vi "PH_HamamatsuCamera.PC set Right.vi"(0 "i ref in":refnum<vi>, 1 "No Info? (False)":bool, 2 "Right":u32, 3 "Maximum Right":u32, 4 "Minimum Right":u32, 5 "error in (no error)":errorcluster, 7 "Right writable? (True)":bool=TRUE) -> (14 "i ref out":refnum<vi>, 17 "Right changed?":bool, 19 "error out":errorcluster)   [LabVIEW 2014]
doc: "This VI sets the incoming value to own attributes and the GUI element."
uses:
  PH_HamamatsuCamera.lvlib
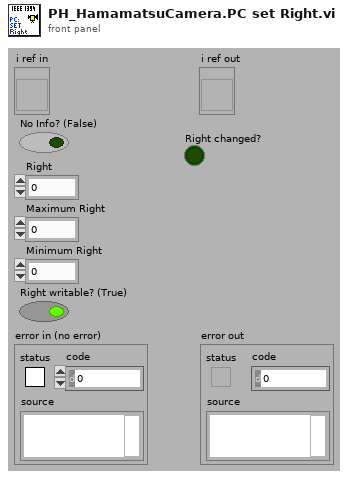
[diagram p1: front panel]
types:
  T1 = enum8{"Enabled", "Disabled", "Disabled and Grayed Out"}
  T2 = typedef "PH_HamamatsuCamera.lvlib/PH_HamamatsuCamera.i attribute.ctl" = cluster{"Gui Refs":cluster{"Frame Rate":refnum<vi>, "Get Frame Rate":refnum<vi>, "Camera State":refnum<vi>, "Start Cam":refnum<vi>, "Show Image":refnum<vi>, "Get Histogram":refnum<vi>, "Mapping":refnum<vi>, "Histogram":refnum<vi>, "Center Cross":refnum<vi>, "Center of Gravity":refnum<vi>, "Scale Factor [%]":refnum<vi>, "Save Image":refnum<vi>, "Palette":refnum<vi>, "Connect":refnum<vi>, "Camera State Bar":refnum<vi>, "Cam Error":refnum<vi>, "Camera Details":refnum<vi>, "ROI":refnum<vi>, "Set ROI to Maximum":refnum<vi>, "Trigger Parameters":refnum<vi>, "Brightness":refnum<vi>, "Shutter":refnum<vi>, "Gain":refnum<vi>, "Trigger Timeout":refnum<vi>, "Subtract Background":refnum<vi>, "Cam List":refnum<vi>, "Parameters":refnum<vi>, "Trigger Polarity":refnum<vi>, "Trigger Mode":refnum<vi>}, "Cam":cluster{"State":T3, "Restart":bool, "Source Notifier":refnum<notifier>, "Handle":i32, "Details":cluster{"Model":string, "Camera ID":string, "Firmware":string}, "Error":errorcluster, "Buffer Info":cluster{"height":u32, "width":u32, "datatype":u32}}, "Images":cluster{"CamI16":T4, "OperationI16":T4, "PSDB I16":T4}, "Window Image":cluster{"Indicate Image":bool, "Window No.":i32, "Scale Facor":dbl, "Center Cross":bool, "Subtract Backgr":bool, "CoG":bool, "Color Palette":cluster{"Red":u8, "Green":u8, "Blue":u8}[], "Image On":bool}, "Default Prdc Int":i32, "Performance":cluster{"on":bool, "Timestamp Last Frame":i32}, "Histogram":cluster{"on":bool, "Mapping":bool}, "Save Image":cluster{"Save":bool, "File refnum":refnum<file>}, "Setting Service ID":i32, "GUI Manager Path":string, "Screen":cluster{"x-resolution":i16, "y-resolution":i16}, "Image Position Path":string, "H Offset":cluster{"Value":i32, "Minimum":i32, "Maximum":i32, "Increment":i32}, "V Offset":cluster{"Value":i32, "Minimum":i32, "Maximum":i32, "Increment":i32}, "H Width":cluster{"Value":i32, "Minimum":i32, "Maximum":i32, "Increment":i32}, "V Width":cluster{"Value":i32, "Minimum":i32, "Maximum":i32, "Increment":i32}, "Trigger Parameters":cluster{"Mode":u32, "Polarity":u32, "Times":u32, "Delay":dbl}, "Trigger Timeout":u32, "Parameters":T5[], "Cam Setting Parameters":cluster{"Brightness":string, "Shutter":string, "Gain":string}}
  T3 = typedef "Device State.ctl" = i32
  T4 = typedef "IMAQ Image.ctl" = refnum<image>
  T5 = typedef "PH_HamamatsuCamera.lvlib/PH_HamamatsuCamera.Parameter Set.ctl" = cluster{"Name":string, "Value":dbl, "Range":cluster{"min":dbl, "max":dbl, "step":dbl}}
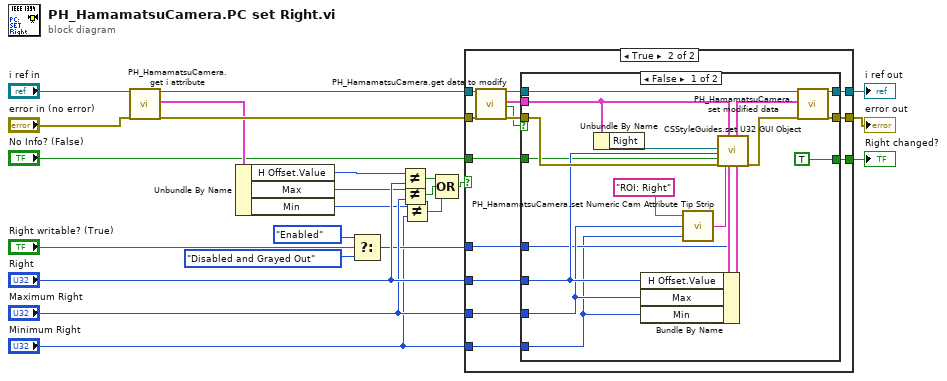
[diagram p0: block diagram]
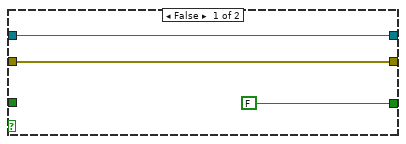
[diagram p2: hidden frame]
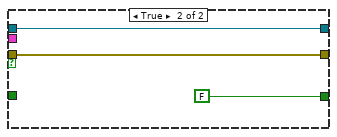
[diagram p3: hidden frame]
diagram:
  n1 = call "PH_HamamatsuCamera.get i attribute.vi"("i ref in"="i ref in", "error in (no error)"="error in (no error)") -> ("i ref out"=w20:refnum<vi>, "i attribute"=w17:T2, "error out"=w18:errorcluster)  [unwired: 15 in]
  n2 = Unbundle By Name(w17) -> ("H Offset.Value"=w16:i32, "Max"=w12:u32, "Min"=w2:u32)
  n3 = Select(t=T1."Enabled" ("Disabled"), s="Right writable? (True)", f=T1."Disabled and Grayed Out" ("Disabled")) -> (s? t:f=w6:T1)
  n4 = Not Equal?(x=w16, y="Right") -> (x != y?=w14:bool)
  n5 = Not Equal?(x=w12, y="Maximum Right") -> (x != y?=w9:bool)
  n6 = Not Equal?(x=w2, y="Minimum Right") -> (x != y?=w3:bool)
  n7 = Compound Arithmetic op=OR(w14, w9, w3) -> (w10:bool)
  n8 = case shown="True" w10 {
    tunnel: [w26 w40] -> w23
    tunnel: [w25 w39] -> w22
    tunnel: w20 -> [w26 w34]
    tunnel: w18 -> [w25 w33]
    tunnel: "Right" -> [_ w32]
    tunnel: [FALSE w31] -> w13
    tunnel: "Maximum Right" -> [_ w30]
    tunnel: "Minimum Right" -> [_ w29]
    tunnel: w6 -> [_ w28]
    tunnel: "No Info? (False)" -> [_ w27]
    frame False {
    }
    frame True {
      n9 = call "PH_HamamatsuCamera.get data to modify.vi"("i ref in"=w34, "error in (no error)"=w33) -> ("i ref out"=w38:refnum<vi>, "i attribute"=w35:T2, "timed out"=w36:bool, "error out"=w37:errorcluster)  [unwired: 14 in]
      n10 = case shown="False" w36 {
        tunnel: [w55 w58] -> w39
        tunnel: [w54 w59] -> w40
        tunnel: w38 -> [w53 w59]
        tunnel: w37 -> [w52 w58]
        tunnel: w35 -> [w50 _]
        tunnel: w32 -> [w47 _]
        tunnel: [TRUE FALSE] -> w31
        tunnel: w30 -> [w44 _]
        tunnel: w29 -> [w41 _]
        tunnel: w28 -> [w43 _]
        tunnel: w27 -> [w42 _]
        frame False {
          n11 = Unbundle By Name(w50) -> ("Right"=w49:refnum<vi>)
          n12 = Bundle By Name(cluster=w50, "H Offset.Value"=w47, "Max"=w44, "Min"=w41) -> (w51:T2)
          n13 = call "PH_HamamatsuCamera.set Numeric Cam Attribute Tip Strip.vi"("Minimum"=w41, "Maximum"=w44, "Attribute"="ROI: Right") -> ("Tip Strip"=w46:string)
          n14 = call "CSStyleGuides.set U32 GUI Object.vi"("U32 Ref"=w49, "Value"=w47, "Blinking (false)"=w42, "error in (no error)"=w52, "Tip Strip [Empty]"=w46, "Disabled (Enabled)"=w43) -> ("error out"=w56:errorcluster)  [unwired: 13 in]
          n15 = call "PH_HamamatsuCamera.set modified data.vi"("i ref in"=w53, "i attribute"=w51, "error in (no error)"=w56) -> ("i ref out"=w54:refnum<vi>, "error out"=w55:errorcluster)  [unwired: 15 in]
        }
        frame True {
        }
      }
    }
  }
  "i ref out" <- w23
  "error out" <- w22
  "Right changed?" <- w13
